vi "Basic Example.vi"() -> ()   [LabVIEW 2020, in "Process.lvclass"]
uses:
  Process.lvclass
panel:
  out "error out":errorcluster
  in  "error in (no error)":errorcluster
  in  "Stop":bool
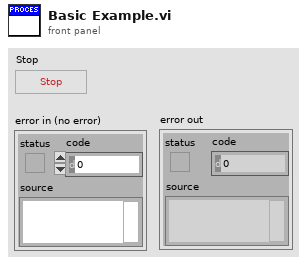
[diagram p1: front panel]
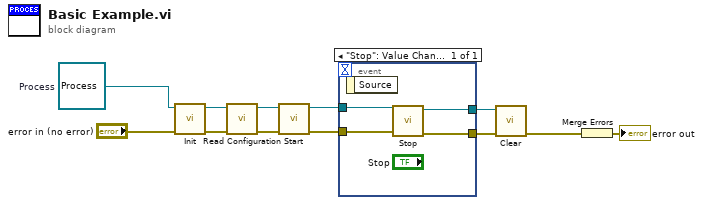
[diagram p0: block diagram]
diagram:
  w1 = refnum<class "Process.lvclass"> refnum  # Process
  n1 = call-dynamic "Init.vi"("error in (no error)"="error in (no error)", "Process In"=w1) -> ("error out"=w3:errorcluster, "Process Out"=w8:refnum<class "Process.lvclass">)  [unwired: 8 in]
  n2 = call-dynamic "Read Configuration.vi"("error in (no error)"=w3, "Process In"=w8) -> ("error out"=w2:errorcluster, "Process Out"=w4:refnum<class "Process.lvclass">)  [unwired: 8 in]
  n3 = call "Start.vi"("error in (no error)"=w2, "Process In"=w4) -> ("error out"=w5:errorcluster, "Process Out"=w6:refnum<class "Process.lvclass">)  [unwired: 8 in]
  n4 = event shown="[0] \"Stop\": Value Change" {
    selector: _ -> [_]
    dyn-events: _ -> [_]
    timeout: _ -> [_]
    tunnel: w6 -> [w16]
    tunnel: [w15] -> w10
    tunnel: w5 -> [w14]
    tunnel: [w13] -> w9
    event "Stop": Value Change {
      n5 = event-data() -> ()  [unwired: 1 in, 1 out]
      n6 = call-dynamic "Stop.vi"("error in (no error)"=w14, "Process In"=w16) -> ("error out"=w13:errorcluster, "Process Out"=w15:refnum<class "Process.lvclass">)  [unwired: 7 in, 1 out]
    }
  }
  n7 = call-dynamic "Clear.vi"("error in (no error)"=w9, "Process In"=w10) -> ("error out"=w11:errorcluster)  [unwired: 8 in, 1 out]
  n8 = Merge Errors(w11) -> (→"error out":errorcluster)
